vi "NI_Mic_Analog.vi"(9 "channel":T1) -> ()   [LabVIEW 2020]
uses:
  <extravilib>/ChannelInstances/Tag-bool/))Channel.ctl
  <extravilib>/ChannelInstances/Tag-bool/Read With Abort.vi
  <extravilib>/ChannelInstances/Tag-bool/EndpointRead.vi
  <extravilib>/ChannelInstances/Tag-bool.lvlib
panel:
  out "Waveform Graph":dynamicdata(graph)
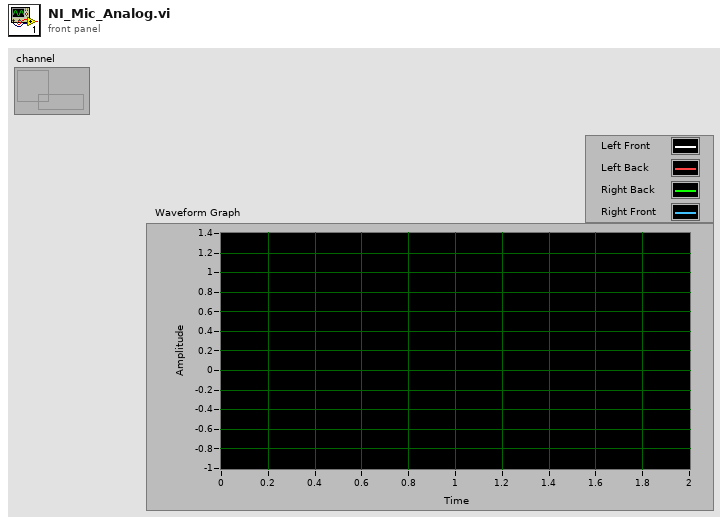
[diagram p1: front panel]
types:
  T1 = typedef "Tag-bool.lvlib/))Channel.ctl" = refnum<queue>
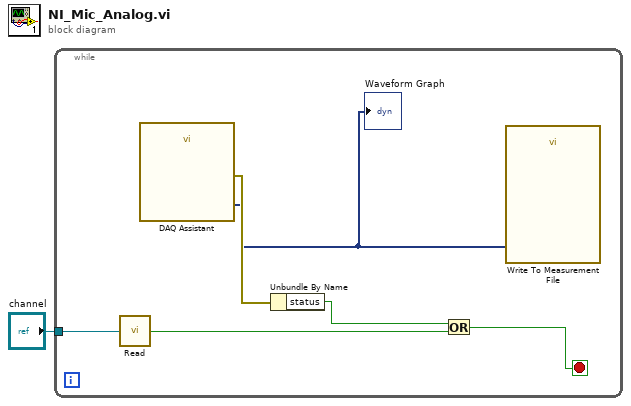
[diagram p0: block diagram]
diagram:
  n1 = while {
    tunnel: "channel" -> [w2]
    stop <- w4 stop-if-true
    n2 = call <extravilib>:"Read.vi"("channel"=w2) -> ("element"=w3:bool)  [unwired: 1 in, 1 out]
    n3 = call "DAQ Assistant"() -> ("data"=w5:dynamicdata, "error out"=w6:errorcluster)  [unwired: 17 in, 1 out]
    "Waveform Graph" <- w5
    n4 = Unbundle By Name(w6) -> ("status"=w7:bool)
    n5 = Or(x=w7, y=w3) -> (x .or. y?=w4:bool)
    n6 = call "Write To Measurement File"("Signals"=w5) -> ()  [unwired: 16 in, 3 out]
  }
